vi "密码登录.vi"(2 "Password":string, 3 "Name":string) -> (0 "Verified":bool, 1 "Name Confirmed":string)   [LabVIEW 2014]
doc: "This VI is the solution to Exercise 1-2 of the LabVIEW Basics II course. \n\nThis VI accepts an employee name and password and searches a table employee information for a match. If a match is found, then the employee is verified, and the employee name is returned."
panel:
  in  "Employee Info Table":string[][](table)=[["20132257", "20132257"], ["20134404", "20134404"], ["", ""], ["", ""]]
  # "* String control *\nLimit to single line enabled"
  # "* String indicator *"
  # "* String control *\nPassword Display enabled\nLimit to single line enabled"
  # "* Round LED *"
  # "* Table *\nRow Headers Visible\nColumn Headers Visible\nCurrent Values Made Default"
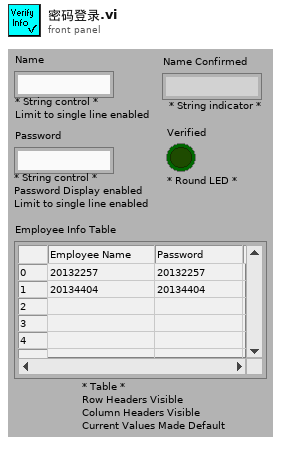
[diagram p1: front panel]
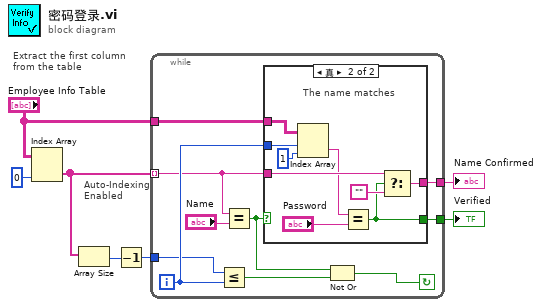
[diagram p0: block diagram]
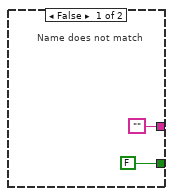
[diagram p2: hidden frame]
diagram:
  # "Extract the first column\nfrom the table"
  # "Auto-Indexing\nEnabled"
  n1 = Index Array "Index Array"(array="Employee Info Table", index (col)=0 ("Disabled Index (col)")) -> (element=w6:string[])  [unwired: 1 in]
  n2 = Array Size(array=w6) -> (size(s)=w5:i32)
  n3 = Decrement(x=w5) -> (x-1=w3:i32)
  n4 = while {
    tunnel: [w12] -> w2
    tunnel: [w16] -> w4
    tunnel: "Employee Info Table" -> [w13]
    tunnel: w3 -> [w10]
    tunnel: w6 -> [w9] mode=indexing
    i -> [w11]
    stop <- w17 continue-if-true
    n5 = Less Or Equal?(x=w10, y=w11) -> (x <= y?=w15:bool)
    n6 = Equal?(x=w9, y="Name") -> (x = y?=w14:bool)
    n7 = case shown="真" w14 {
      tunnel: w11 -> [_ w28]
      tunnel: [FALSE w24] -> w16
      tunnel: w13 -> [_ w26]
      tunnel: ["" w23] -> w12
      tunnel: w9 -> [_ w22]
      frame False {
        # "Name does not match"
      }
      frame True {
        # "The name matches"
        n8 = Index Array "Index Array"(array=w26, index (row)=w28, index (col)=1 ("Disabled Index (col)")) -> (element=w21:string)
        n9 = Equal?(x=w21, y="Password") -> (x = y?=w24:bool)
        n10 = Select(t=w22, s=w24, f="") -> (s? t:f=w23:string)
      }
    }
    n11 = Not Or(1:w15, 2:w14) -> (0:w17:bool)
  }
  "Verified" <- w4
  "Name Confirmed" <- w2
